vi "Enable Controls.vi"(8 "error in (no error)":errorcluster, 10 "Disabled":T1(ring), 11 "Server in":refnum<class "Server.lvclass">) -> (0 "error out":errorcluster, 3 "Server out":refnum<class "Server.lvclass">)   [LabVIEW 2020, in "Server.lvlib" / "Server.lvclass"]
uses:
  Server.lvclass
  Server.lvclass/Server.ctl
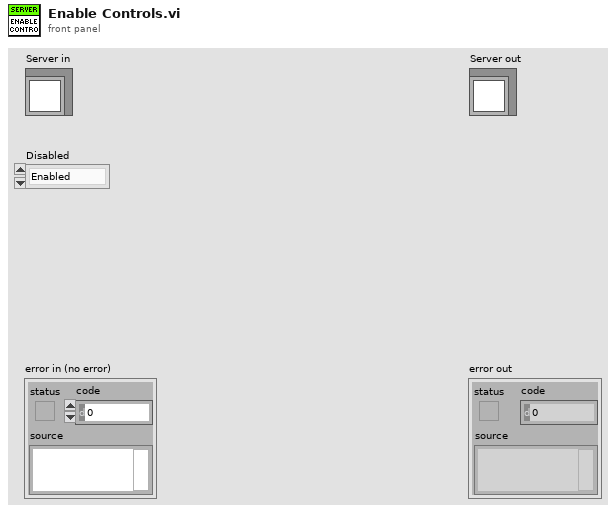
[diagram p1: front panel]
types:
  T1 = enum8{"Enabled", "Disabled", "Disabled and Grayed Out"}
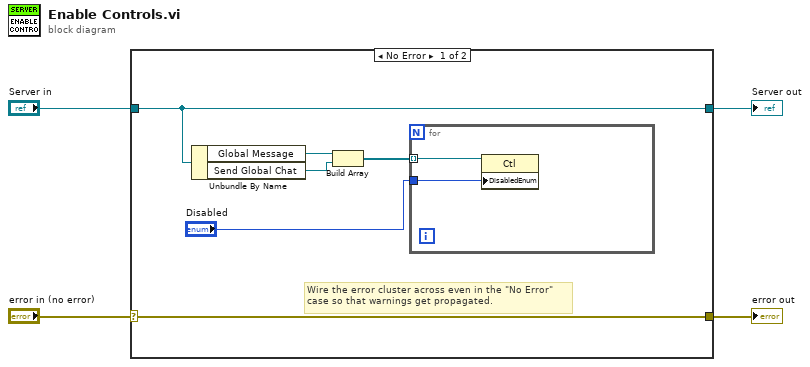
[diagram p0: block diagram]
diagram:
  n1 = case shown="No Error" "error in (no error)" {
    selector: "error in (no error)" -> [w10 w14]
    tunnel: [w10 w14] -> w3
    tunnel: [w9 w13] -> w1
    tunnel: "Server in" -> [w9 w13]
    frame No Error {
      # "Wire the error cluster across even in the \"No Error\"\ncase so that warnings get propagated."
      n2 = Unbundle By Name(w9) -> ("Global Message"=w8:refnum<vi>, "Send Global Chat"=w7:refnum<vi>)
      n3 = Build Array(w8, w7) -> (w6:refnum<vi>[])
      n4 = for {
        tunnel: w6 -> [w12] mode=indexing
        tunnel: "Disabled" -> [w11]
        n5 = property class="Ctl"(reference=w12, "DisabledEnum"=w11) -> ()  [unwired: 1 in, 2 out]
      }
    }
    frame Error {
    }
  }
  "error out" <- w3
  "Server out" <- w1
